vi "Reload Previous Commands.vi"(6 "Front (T) Back (F)":bool, 8 "error in (no error)":errorcluster, 9 "length":i32, 10 "index":i32, 11 "Command Handler in":refnum<class "Command Handler.lvclass">) -> (0 "error out":errorcluster, 3 "Command Handler out":refnum<class "Command Handler.lvclass">)   [LabVIEW 2017, in "Command Handler.lvlib" / "Command Handler.lvclass"]
uses:
  Command Handler.lvclass
  Command Handler.lvclass/Command Handler.ctl
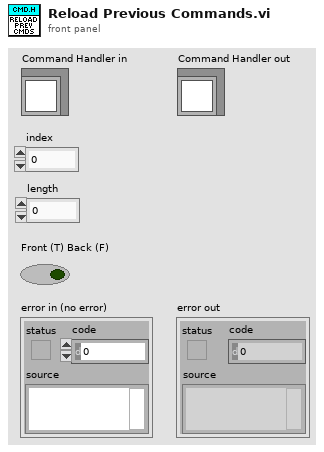
[diagram p1: front panel]
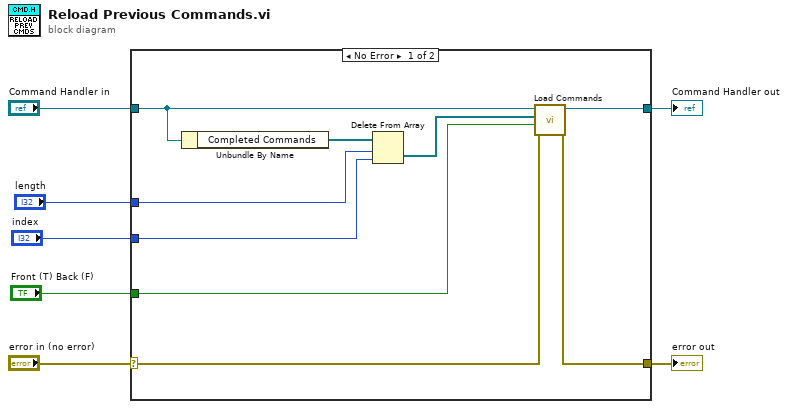
[diagram p0: block diagram]
diagram:
  n1 = case shown="No Error" "error in (no error)" {
    selector: "error in (no error)" -> [w12 w18]
    tunnel: [w11 w18] -> w6
    tunnel: [w13 w17] -> w4
    tunnel: "Command Handler in" -> [w14 w17]
    tunnel: "index" -> [w15 _]
    tunnel: "Front (T) Back (F)" -> [w9 _]
    tunnel: "length" -> [w8 _]
    frame No Error {
      n2 = Unbundle By Name(w14) -> ("Completed Commands"=w16:refnum<class "Command.lvclass">[])
      n3 = Delete From Array(array=w16, length=w8, index=w15) -> (deleted portion=w10:refnum<class "Command.lvclass">[])  [unwired: 1 out]
      n4 = call-dynamic "Load Commands.vi"("error in (no error)"=w12, "Front (T) Back (F)"=w9, "Commands In"=w10, "Command Handler in"=w14) -> ("error out"=w11:errorcluster, "Command Handler out"=w13:refnum<class "Command Handler.lvclass">)  [unwired: 6 in]
    }
    frame Error {
    }
  }
  "error out" <- w6
  "Command Handler out" <- w4
